vi "CreateFakeTestSuite.vi"(8 "error in (no error)":errorcluster, 10 "Name":string) -> (0 "error out":errorcluster, 3 "FakeTestSuite out":refnum<class "FakeTestSuite.lvclass">)   [LabVIEW 2017, in "ResultTreeListener.Tests.lvlib" / "Support.lvlib" / "FakeTestSuite.lvclass"]
uses:
  FakeTestSuite.lvclass
  FakeTestSuite.lvclass/FakeTestSuite.ctl
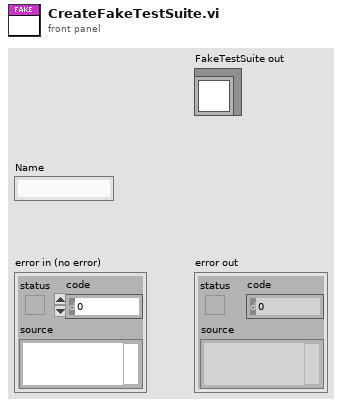
[diagram p1: front panel]
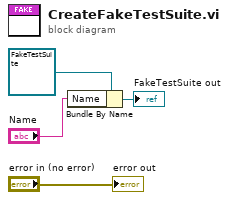
[diagram p0: block diagram]
diagram:
  n1 = Bundle By Name(cluster=refnum<class "FakeTestSuite.lvclass"> refnum ("FakeTestSuite in"), "Name"="Name") -> (→"FakeTestSuite out":refnum<class "FakeTestSuite.lvclass">)
  "error out" <- "error in (no error)"
